vi "Launcher.vi"() -> ()   [LabVIEW 2020]
uses:
  UI Actor.lvclass
  C:/Program Files (x86)/National Instruments/LabVIEW 2020/vi.lib/ActorFramework/Actor/Actor.lvclass
  Implementation/Arduino/Arduino.lvclass
  Implementation/NXP/NXP.lvclass
  Implementation/Simulated Device/Simulated Device.lvclass
  UI Actor.lvclass/UI Actor.ctl
  Write Serial Device.lvclass.vi
  Write VISA resource name.vi
  <vilib>/ActorFramework/Actor/Actor.lvclass
panel:
  in  "COM PORT":refnum<visa-resource-name>
  in  "Microcontrollers":enum16{"Arduino", "NXP", "Simulado"}(ring)
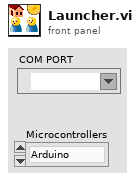
[diagram p1: front panel]
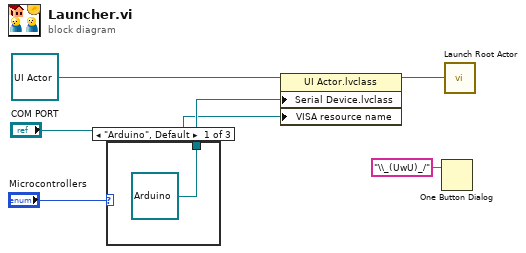
[diagram p0: block diagram]
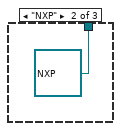
[diagram p2: hidden frame]
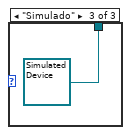
[diagram p3: hidden frame]
diagram:
  n1 = case shown="\"Arduino\", Default" "Microcontrollers" {
    tunnel: [refnum<class "Arduino.lvclass"> refnum ("Arduino.lvclass") refnum<class "NXP.lvclass"> refnum ("NXP.lvclass") refnum<class "Simulated Device.lvclass"> refnum ("Simulated Device.lvclass")] -> w3
    frame "Arduino", Default {
    }
    frame "NXP" {
    }
    frame "Simulado" {
    }
  }
  n2 = property class="UI Actor.lvclass"(reference=refnum<class "UI Actor.lvclass"> refnum ("UI Actor.lvlib:UI Actor.lvclass"), "Serial Device.lvclass"=w3, "VISA resource name"="COM PORT") -> (reference out=w4:refnum<class "UI Actor.lvclass">)  [unwired: 1 in, 1 out]
  n3 = One Button Dialog(message="\\_(UwU)_/") -> ()  [unwired: 1 in, 1 out]
  n4 = call <vilib>:"Launch Root Actor.vi"("Actor"=w4) -> ()  [unwired: 9 in, 2 out]
